vi "cluster creator.vi"() -> ()   [LabVIEW 2017]
panel:
  out "cluster":T1
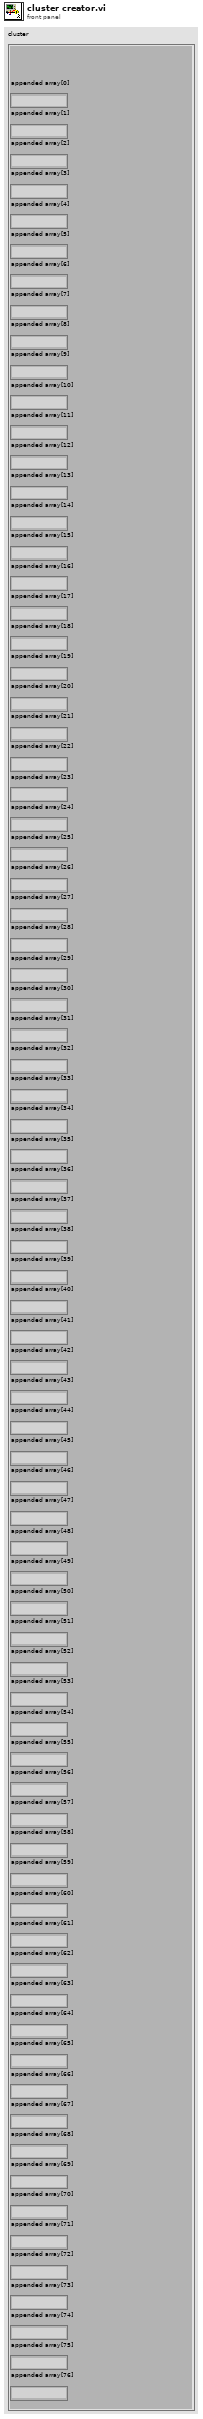
[diagram p1: front panel]
types:
  T1 = cluster{"appended array[0]":string, "appended array[1]":string, "appended array[2]":string, "appended array[3]":string, "appended array[4]":string, "appended array[5]":string, "appended array[6]":string, "appended array[7]":string, "appended array[8]":string, "appended array[9]":string, "appended array[10]":string, "appended array[11]":string, "appended array[12]":string, "appended array[13]":string, "appended array[14]":string, "appended array[15]":string, "appended array[16]":string, "appended array[17]":string, "appended array[18]":string, "appended array[19]":string, "appended array[20]":string, "appended array[21]":string, "appended array[22]":string, "appended array[23]":string, "appended array[24]":string, "appended array[25]":string, "appended array[26]":string, "appended array[27]":string, "appended array[28]":string, "appended array[29]":string, "appended array[30]":string, "appended array[31]":string, "appended array[32]":string, "appended array[33]":string, "appended array[34]":string, "appended array[35]":string, "appended array[36]":string, "appended array[37]":string, "appended array[38]":string, "appended array[39]":string, "appended array[40]":string, "appended array[41]":string, "appended array[42]":string, "appended array[43]":string, "appended array[44]":string, "appended array[45]":string, "appended array[46]":string, "appended array[47]":string, "appended array[48]":string, "appended array[49]":string, "appended array[50]":string, "appended array[51]":string, "appended array[52]":string, "appended array[53]":string, "appended array[54]":string, "appended array[55]":string, "appended array[56]":string, "appended array[57]":string, "appended array[58]":string, "appended array[59]":string, "appended array[60]":string, "appended array[61]":string, "appended array[62]":string, "appended array[63]":string, "appended array[64]":string, "appended array[65]":string, "appended array[66]":string, "appended array[67]":string, "appended array[68]":string, "appended array[69]":string, "appended array[70]":string, "appended array[71]":string, "appended array[72]":string, "appended array[73]":string, "appended array[74]":string, "appended array[75]":string, "appended array[76]":string}
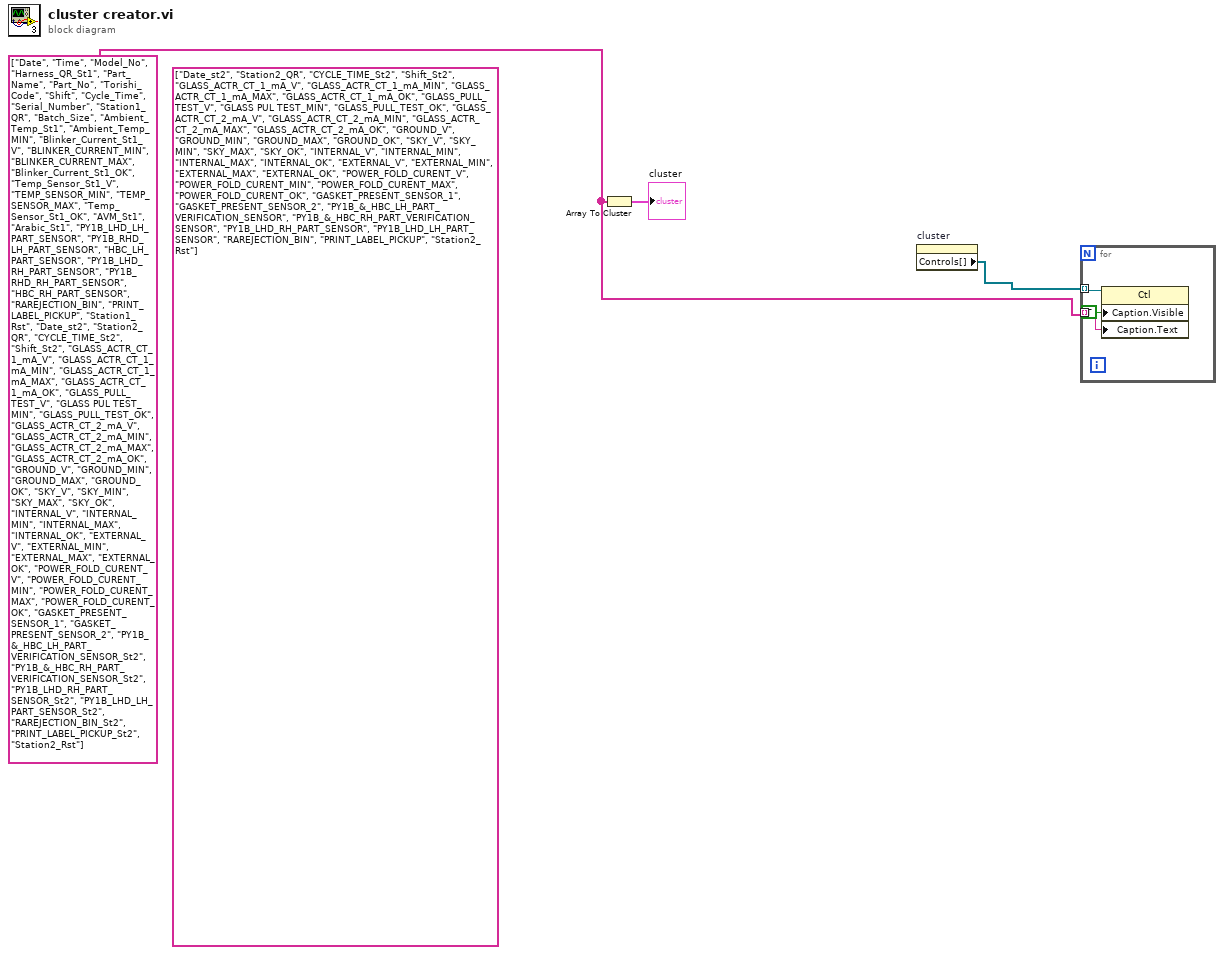
[diagram p0: block diagram]
diagram:
  w3 = string[] ["Date", "Time", "Model_No", "Harness_QR_St1", "Part_Name", "Part_No", "Torishi_Code", "Shift", "Cycle_Time", "Serial_Number", "Station1_QR", "Batch_Size", "Ambient_Temp_St1", "Ambient_Temp_MIN", "Blinker_Current_St1_V", "BLINKER_CURRENT_MIN", "BLINKER_CURRENT_MAX", "Blinker_Current_St1_OK", "Temp_Sensor_St1_V", "TEMP_SENSOR_MIN", "TEMP_SENSOR_MAX", "Temp_Sensor_St1_OK", "AVM_St1", "Arabic_St1", "PY1B_LHD_LH_PART_SENSOR", "PY1B_RHD_LH_PART_SENSOR", "HBC_LH_PART_SENSOR", "PY1B_LHD_RH_PART_SENSOR", "PY1B_RHD_RH_PART_SENSOR", "HBC_RH_PART_SENSOR", "RAREJECTION_BIN", "PRINT_LABEL_PICKUP", "Station1_Rst", "Date_st2", "Station2_QR", "CYCLE_TIME_St2", "Shift_St2", "GLASS_ACTR_CT_1_mA_V", "GLASS_ACTR_CT_1_mA_MIN", "GLASS_ACTR_CT_1_mA_MAX", "GLASS_ACTR_CT_1_mA_OK", "GLASS_PULL_TEST_V", "GLASS PUL TEST_MIN", "GLASS_PULL_TEST_OK", "GLASS_ACTR_CT_2_mA_V", "GLASS_ACTR_CT_2_mA_MIN", "GLASS_ACTR_CT_2_mA_MAX", "GLASS_ACTR_CT_2_mA_OK", "GROUND_V", "GROUND_MIN", "GROUND_MAX", "GROUND_OK", "SKY_V", "SKY_MIN", "SKY_MAX", "SKY_OK", "INTERNAL_V", "INTERNAL_MIN", "INTERNAL_MAX", "INTERNAL_OK", "EXTERNAL_V", "EXTERNAL_MIN", "EXTERNAL_MAX", "EXTERNAL_OK", "POWER_FOLD_CURENT_V", "POWER_FOLD_CURENT_MIN", "POWER_FOLD_CURENT_MAX", "POWER_FOLD_CURENT_OK", "GASKET_PRESENT_SENSOR_1", "GASKET_PRESENT_SENSOR_2", "PY1B_&_HBC_LH_PART_VERIFICATION_SENSOR_St2", "PY1B_&_HBC_RH_PART_VERIFICATION_SENSOR_St2", "PY1B_LHD_RH_PART_SENSOR_St2", "PY1B_LHD_LH_PART_SENSOR_St2", "RAREJECTION_BIN_St2", "PRINT_LABEL_PICKUP_St2", "Station2_Rst"] ("appended array")
  (unwired) string[] ["Date_st2", "Station2_QR", "CYCLE_TIME_St2", "Shift_St2", "GLASS_ACTR_CT_1_mA_V", "GLASS_ACTR_CT_1_mA_MIN", "GLASS_ACTR_CT_1_mA_MAX", "GLASS_ACTR_CT_1_mA_OK", "GLASS_PULL_TEST_V", "GLASS PUL TEST_MIN", "GLASS_PULL_TEST_OK", "GLASS_ACTR_CT_2_mA_V", "GLASS_ACTR_CT_2_mA_MIN", "GLASS_ACTR_CT_2_mA_MAX", "GLASS_ACTR_CT_2_mA_OK", "GROUND_V", "GROUND_MIN", "GROUND_MAX", "GROUND_OK", "SKY_V", "SKY_MIN", "SKY_MAX", "SKY_OK", "INTERNAL_V", "INTERNAL_MIN", "INTERNAL_MAX", "INTERNAL_OK", "EXTERNAL_V", "EXTERNAL_MIN", "EXTERNAL_MAX", "EXTERNAL_OK", "POWER_FOLD_CURENT_V", "POWER_FOLD_CURENT_MIN", "POWER_FOLD_CURENT_MAX", "POWER_FOLD_CURENT_OK", "GASKET_PRESENT_SENSOR_1", "GASKET_PRESENT_SENSOR_2", "PY1B_&_HBC_LH_PART_VERIFICATION_SENSOR", "PY1B_&_HBC_RH_PART_VERIFICATION_SENSOR", "PY1B_LHD_RH_PART_SENSOR", "PY1B_LHD_LH_PART_SENSOR", "RAREJECTION_BIN", "PRINT_LABEL_PICKUP", "Station2_Rst"] ("columns")
  n1 = Array To Cluster(array=w3) -> (cluster=→"cluster":T1)
  n2 = property on="cluster" class="Clust (strict)"() -> ("Controls[]"=w1:refnum<vi>[])  [unwired: 2 in, 2 out]
  n3 = for {
    tunnel: w1 -> [w6] mode=indexing
    tunnel: w3 -> [w5] mode=indexing
    n4 = property class="Ctl"(reference=w6, "Caption.Visible"=TRUE, "Caption.Text"=w5) -> ()  [unwired: 1 in, 2 out]
  }
